vi "Format_ACAnalysis.vi"(6 "CMRR":ext, 8 "PGA":i32, 9 "ACParameter":T1, 11 "AC Analysis [] in":string[][](array[string])) -> (3 "AC Analysis [] out":string[][](array[string]))   [LabVIEW 2010]
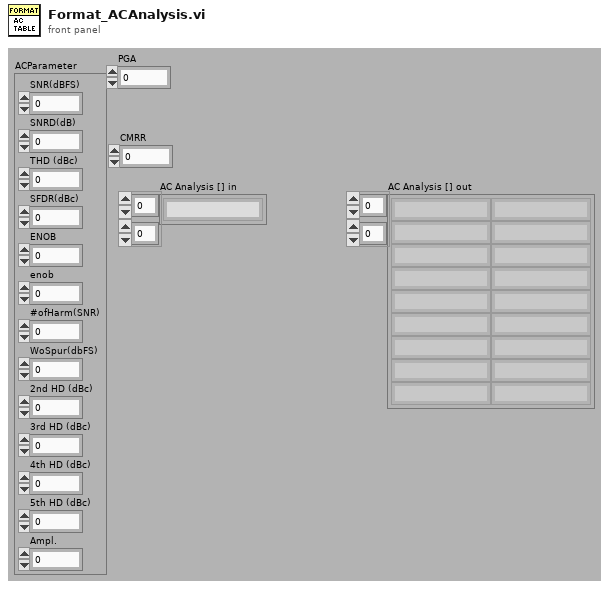
[diagram p1: front panel]
types:
  T1 = cluster{"SNR(dBFS)":dbl, "SNRD(dB)":dbl, "THD (dBc)":dbl, "SFDR(dBc)":dbl, "ENOB":dbl, "enob":dbl, "#ofHarm(SNR)":dbl, "WoSpur(dbFS)":dbl, "2nd HD (dBc)":dbl, "3rd HD (dBc)":dbl, "4th HD (dBc)":dbl, "5th HD (dBc)":dbl, "Ampl.":dbl}
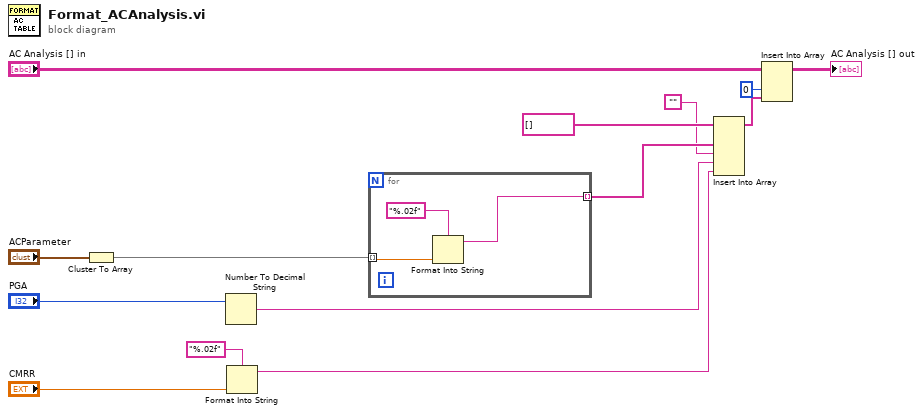
[diagram p0: block diagram]
diagram:
  n1 = Cluster To Array(cluster="ACParameter") -> (array=w13:dbl[])
  n2 = Number To Decimal String(number="PGA") -> (decimal integer string=w1:string)  [unwired: 1 out]
  n3 = Format Into String(format string="%.02f", "CMRR") -> (resulting string=w3:string)  [unwired: 2 in, 1 out]
  n4 = for {
    tunnel: w13 -> [w17] mode=indexing
    tunnel: [w15] -> w5 mode=indexing
    n5 = Format Into String(format string="%.02f", w17) -> (resulting string=w15:string)  [unwired: 2 in, 1 out]
  }
  n6 = Insert Into Array(array=string[] [], new element #1=w5, new element #2="", new element #3=w1, new element #4=w3) -> (w7:string[])  [unwired: 1 in]
  n7 = Insert Into Array(array="AC Analysis [] in", index (col)=0 ("disabled index (col)"), new element=w7) -> (→"AC Analysis [] out":string[][])  [unwired: 1 in]
